vi "test_python_pattern.vi"() -> ()   [LabVIEW 2011]
uses:
  Periodic Spot Pattern Parameters.ctl
  Periodic Spot Pattern Parameters2.ctl
panel:
  out "error out 2":errorcluster
  out "Float Matrix":dbl[][](array[numeric])
  in  "Pattern Definition":T1={"Spot pitch (pixels)"=23.1, "Tilt Angle (deg)"=0.0, "Horizontal Offset (pixels)"=91.9, "Vertical Offset (pixels)"=14.1, "# Horizontal Spots"=8, "# Vertical Spots"=1, "Spot size (pixels)"=23.1, "Darken center spot"=FALSE, "Exact Phase Formula"=TRUE, "phase wrapping"=FALSE, "Set Focus (mm)"=32.0, "Add phase"=4.0, "phase_factor"=65.0, "Steering LW"=2.0, "Steering vmax"=0.0, "phase_overshoot"=TRUE, "Focal shift param"=0.0, "x0 focal shift"=0.0, "y0 focal shift"=0.0, "hv_steering"=TRUE, "fixed"=TRUE, "Pad"=0.0, "dark_all"=FALSE, "nospot"=FALSE, "Laser wavelength"=6.28e-07} {"Laser wavelength" min=0.0 max=500.0 format="%^#.3e"; "Pad" min=0.0 max=500.0 step=1.0 format="%#.0g"; "y0 focal shift" min=0.0 max=500.0 format="%#.3g"; "x0 focal shift" min=0.0 max=500.0 format="%#.3g"; "Focal shift param" min=0.0 max=500.0 format="%#.3g"; "Steering vmax" min=0.0 max=500.0 format="%#.3g"; "Steering LW" min=0.0 max=500.0 format="%#.3g"; "phase_factor" min=0.0 max=500.0 format="%#.3f"; "Add phase" min=0.0 max=500.0 format="%#.3f"; "Set Focus (mm)" min=0.0 max=500.0 format="%#.3g"; "Spot size (pixels)" min=1.0 format="%.2g"; "# Vertical Spots" min=1 step=1; "# Horizontal Spots" min=1 step=1; "Vertical Offset (pixels)" format="%.2f"; "Horizontal Offset (pixels)" format="%.2f"; "Tilt Angle (deg)" min=-90.0 max=90.0 format="%.2g"; "Spot pitch (pixels)" min=1.0 format="%.2g"}
  out "error out":errorcluster
  in  "error in (no error)":errorcluster
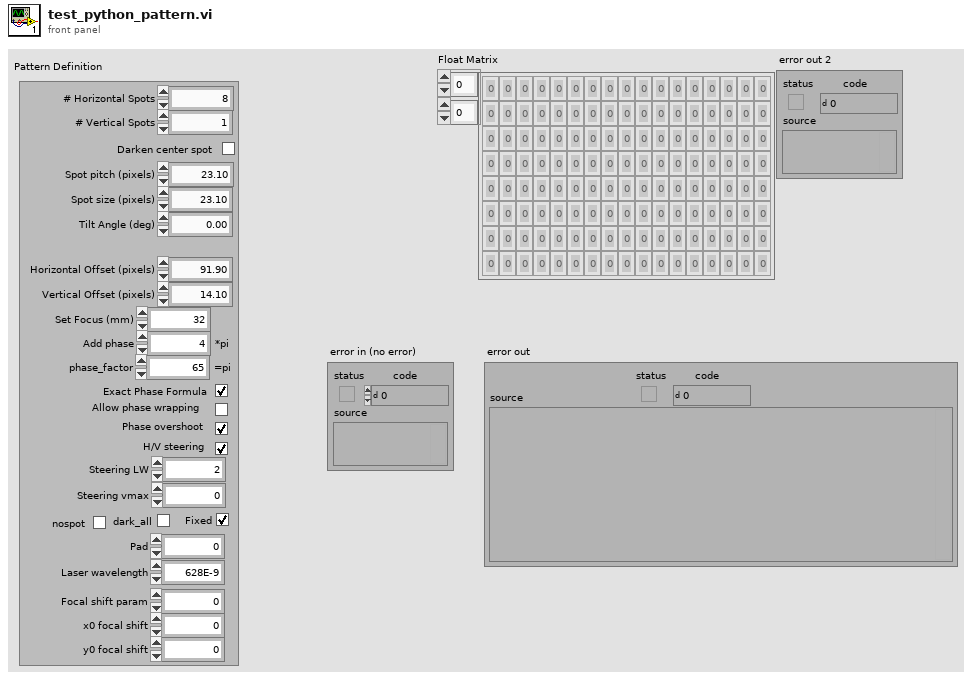
[diagram p1: front panel]
types:
  T1 = typedef "Periodic Spot Pattern Parameters.ctl" = cluster{"Spot pitch (pixels)":dbl, "Tilt Angle (deg)":dbl, "Horizontal Offset (pixels)":dbl, "Vertical Offset (pixels)":dbl, "# Horizontal Spots":u32, "# Vertical Spots":u32, "Spot size (pixels)":dbl, "Darken center spot":bool, "Exact Phase Formula":bool, "phase wrapping":bool, "Set Focus (mm)":T2, "Add phase":dbl, "phase_factor":dbl, "Steering LW":T2, "Steering vmax":T2, "phase_overshoot":bool, "Focal shift param":T2, "x0 focal shift":T2, "y0 focal shift":T2, "hv_steering":bool, "fixed":bool, "Pad":T2, "dark_all":bool, "nospot":bool, "Laser wavelength":dbl}
  T2 = typedef "Periodic Spot Pattern Parameters2.ctl" = dbl
  T3 = typedef "PYTHON Session Refnum__ogtk.ctl" = refnum<k1>
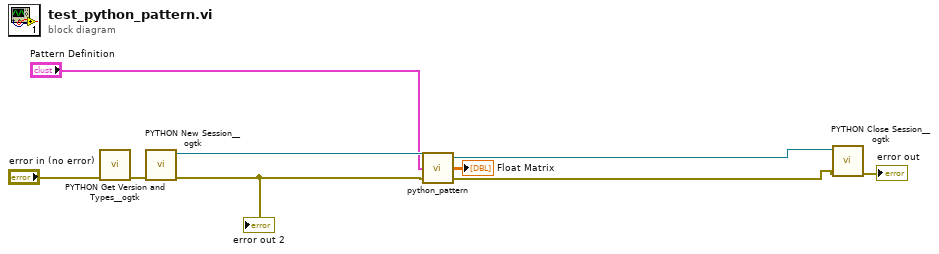
[diagram p0: block diagram]
diagram:
  n1 = call <userlib>:"PYTHON Get Version and Types__ogtk.vi"("error in (no error)"="error in (no error)") -> ("error out"=w9:errorcluster)  [unwired: 4 in, 2 out]
  n2 = call <userlib>:"PYTHON New Session__ogtk.vi"("error in (no error)"=w9) -> ("error out"=w5:errorcluster, "Python Session"=w6:T3)  [unwired: 5 in]
  "error out 2" <- w5
  n3 = call "python_pattern.vi"("Python error in"=w5, "Pattern Definition"="Pattern Definition", "Python Session in"=w6) -> ("Python error out"=w3:errorcluster, "Float Matrix"=→"Float Matrix":dbl[][], "Python Session out"=w4:T3)
  n4 = call <userlib>:"PYTHON Close Session__ogtk.vi"("error in (no error)"=w3, "Python Session in"=w4) -> ("error out"=→"error out":errorcluster)  [unwired: 5 in]
